vi "XML ( Set Node Value ).vi"   [LabVIEW 2018, in "XML.lvlib" / "XML.lvclass"]
uses:
  XML.lvclass
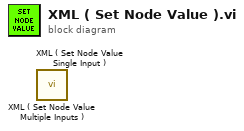
[diagram p0: block diagram]
diagram:
  n1 = call "XML ( Set Node Value Multiple Inputs ).vi"() -> ()  [unwired: 10 in, 2 out]
  n2 = call "XML ( Set Node Value Single Input ).vi"() -> ()  [unwired: 10 in, 2 out]
